vi "PM100D_SetRngIndex.vi"(5 "VISAin":refnum<visa-resource-name>, 7 "Unit":string, 9 "AUTO":bool, 11 "error in":errorcluster, 12 "SensType":i32, 13 "Rng_Array":string[](array[string]), 14 "Index":i32) -> (4 "VISAout":refnum<visa-resource-name>, 6 "lblRange":string, 8 "Numeric 2":dbl, 10 "AUTO?":bool, 15 "error out 2":errorcluster)   [LabVIEW 2009]
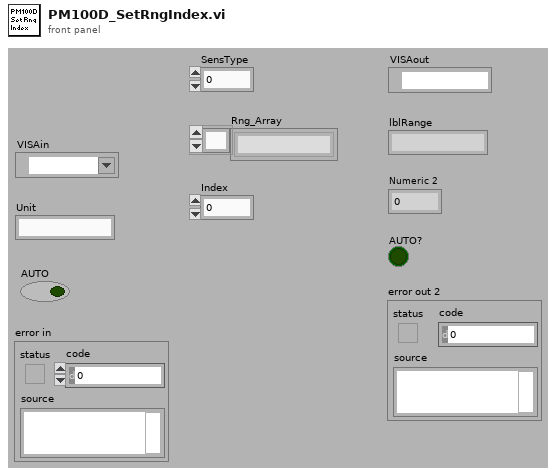
[diagram p1: front panel]
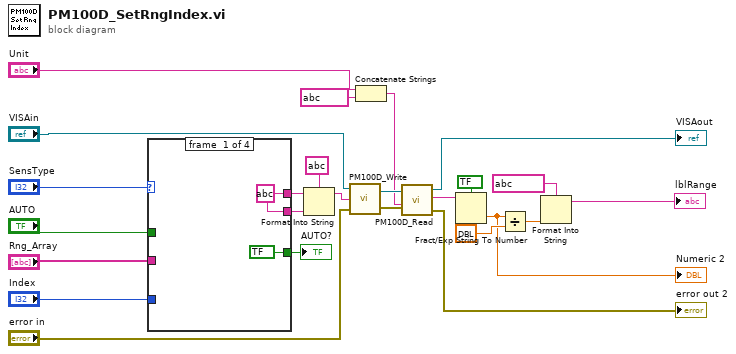
[diagram p0: block diagram]
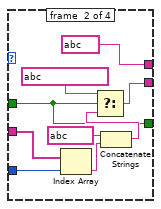
[diagram p2: hidden frame]
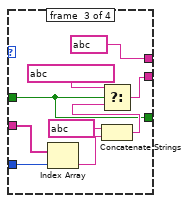
[diagram p3: hidden frame]
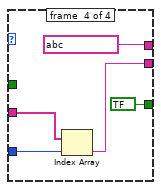
[diagram p4: hidden frame]
diagram:
  n1 = case shown="2" "SensType" {
    tunnel: [w27 string ? string ? string ? ("string")] -> w10
    tunnel: "Index" -> [_ w36 w45 w50]
    tunnel: "AUTO" -> [_ w28 w37 _]
    tunnel: [w27 w34 w43 w49] -> w12
    tunnel: "Rng_Array" -> [_ w33 w42 w48]
    tunnel: [bool ? ("AUTO") w28 w37 bool ? ("AUTO")] -> w22
    frame #0 {
      w27 = string ?
    }
    frame #1 {
      n2 = Index Array(array=w33, index=w36) -> (element=w32:string)
      n3 = Concatenate Strings(string ? ("string"), w32) -> (w30:string)
      n4 = Select(t=string ?, s=w28, f=w30) -> (s? t:f=w34:string)
    }
    frame #2 {
      n5 = Index Array(array=w42, index=w45) -> (element=w39:string)
      n6 = Concatenate Strings(string ? ("string"), w39) -> (w38:string)
      n7 = Select(t=string ?, s=w37, f=w38) -> (s? t:f=w43:string)
    }
    frame #3 {
      n8 = Index Array(array=w48, index=w50) -> (element=w49:string)
    }
  }
  "AUTO?" <- w22
  n9 = Format Into String(format string=string ?, initial string=w10, w12) -> (resulting string=w9:string)  [unwired: 1 in, 1 out]
  n10 = call "PM100D_Write.vi"("error in (no error)"="error in", "Command"=w9, "VISA in"="VISAin") -> ("error out"=w20:errorcluster, "VISA out"=w21:refnum<visa-resource-name>)
  n11 = Concatenate Strings("Unit", string ? ("string")) -> (w13:string)
  n12 = call "PM100D_Read.vi"("error in (no error)"=w20, "Command"=w13, "VISA in"=w21) -> ("error out"=→"error out 2":errorcluster, "ReadValue"=w3:string, "VISA out"=→"VISAout":refnum<visa-resource-name>)  [unwired: 1 in]
  n13 = Fract/Exp String To Number(use system decimal point (T)=bool ?, string=w3) -> (number=w5:dbl)  [unwired: 2 in, 1 out]
  "Numeric 2" <- w5
  n14 = Divide(x=w5, y=dbl ?) -> (x/y=w7:dbl)
  n15 = Format Into String(format string=string ?, w7) -> (resulting string=→"lblRange":string)  [unwired: 2 in, 1 out]
